vi "DAQ Close.vi"(8 "error in (no error)":errorcluster caption="错误输入（无错误）", 11 "DAQ Task":refnum<k21> caption="DAQ任务") -> (0 "error out":errorcluster caption="错误输出")   [LabVIEW 2013]
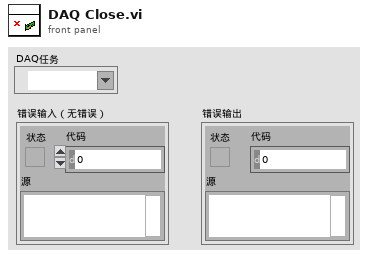
[diagram p1: front panel]
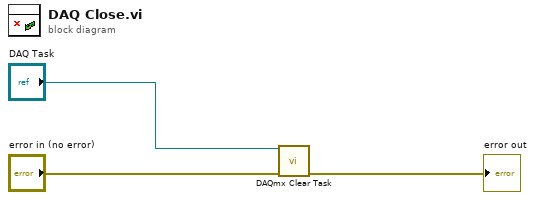
[diagram p0: block diagram]
diagram:
  n1 = call <vilib>:"DAQmx Clear Task.vi"("task in"="DAQ Task", "error in"="error in (no error)") -> ("error out"=→"error out":errorcluster)  [unwired: 13 in]
